vi "Pre Launch Init.vi"(11 "Topic in":refnum<class "Topic.lvclass">) -> (0 "error out":errorcluster, 3 "Topic out":refnum<class "Topic.lvclass">)   [LabVIEW 2017, in "Mediator.lvlib" / "Topic.lvclass"]
doc: "(<B>Filename</B>: Actor Framework.lvlib:Actor.lvclass:Pre Launch Init.vi)\n\nDefines behavior that occurs after the Launch Nested Actor method is invoked but before the actor's Actor Core method begins running.\n\nBy default, this method does nothing. A descendant class may override it to define behavior."
uses:
  Topic.lvclass
  <vilib>/ActorFramework/Actor/Actor.lvclass
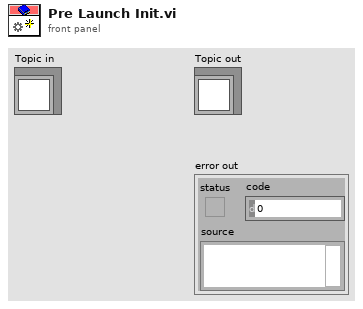
[diagram p1: front panel]
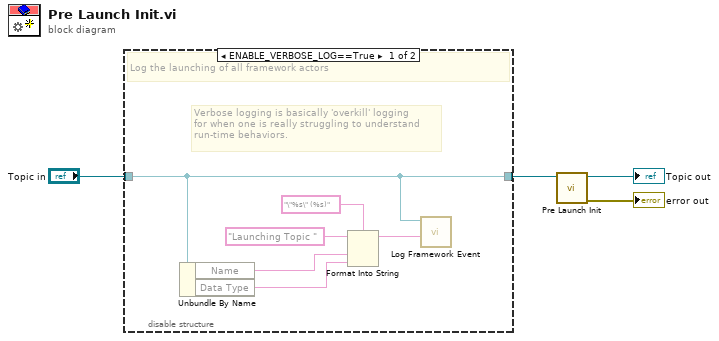
[diagram p0: block diagram]
diagram:
  n1 = disable-structure shown="ENABLE_VERBOSE_LOG==True" {
    disable-tunnel: "Topic in" -> [w10 w11]
    disable-tunnel: [w10 w11] -> w2
    frame condition #0 {
      # "Verbose logging is basically 'overkill' logging\nfor when one is really struggling to understand\nrun-time behaviors."
      # "Log the launching of all framework actors"
      n2 = Unbundle By Name(w10) -> ("Name"=w8:string, "Data Type"=w7:string)
      n3 = Format Into String(format string="\"%s\" (%s)", initial string="Launching Topic " ("Data To Log"), w8, w7) -> (resulting string=w5:string)  [unwired: 1 in, 1 out]
      n4 = call "Log Framework Event.vi"("Data To Log"=w5, "Topic In"=w10) -> ()  [unwired: 9 in, 1 out]
    }
    frame condition #1 (active) {
      # "Remove all logging from this method at compile time"
    }
  }
  n5 = call-parent "Pre Launch Init.vi"("Actor in"=w2) -> ("error out"=→"error out":errorcluster, "Actor out"=→"Topic out":refnum<class "Topic.lvclass">)  [unwired: 9 in]
